vi "Auto Drive v2.vi"(9 "Orientation Angle":dbl, 10 "Move Distance":dbl, 11 "Movement Angle":dbl) -> (0 "Done Moving":bool)   [LabVIEW 2017]
uses:
  Robot Global Data.vi
  <vilib>/addons/control/pid/pid.llb/PID (DBL).vi
  <vilib>/addons/control/pid/NI_PID_pid.lvlib
panel:
  out "Last 25 Compare Values":bool[](array[boolean])
  out "Drive Speed":enum16{"Fast", "Slow", "Approach", "Stopping"}(ring)
  in  "Stopping Setpoint":dbl=0.1
  in  "Approach Setpoint":dbl=0.3
  in  "Slow Setpoint":dbl=0.5
  in  "Allowable Encoder Error":dbl=425.0
  out "Encoder Out":dbl
  in  "Encoder":dbl
  out "Drive Encoder Value":dbl(graph)
  out "output - Angle":dbl(graph)
  in  "PID gains - Angle":T1={"proportional gain (Kc)"=0.0012, "integral time (Ti, min)"=0.0, "derivative time (Td, min)"=0.0002} {"derivative time (Td, min)" step=0.001 format="%.5f"; "integral time (Ti, min)" step=0.001 format="%.5f"; "proportional gain (Kc)" step=0.001 format="%.5f"}
  # "Note: Setpoint Values\nare based on decimal\nprecentages. Ex. 80%\nwill be entered 0.8"
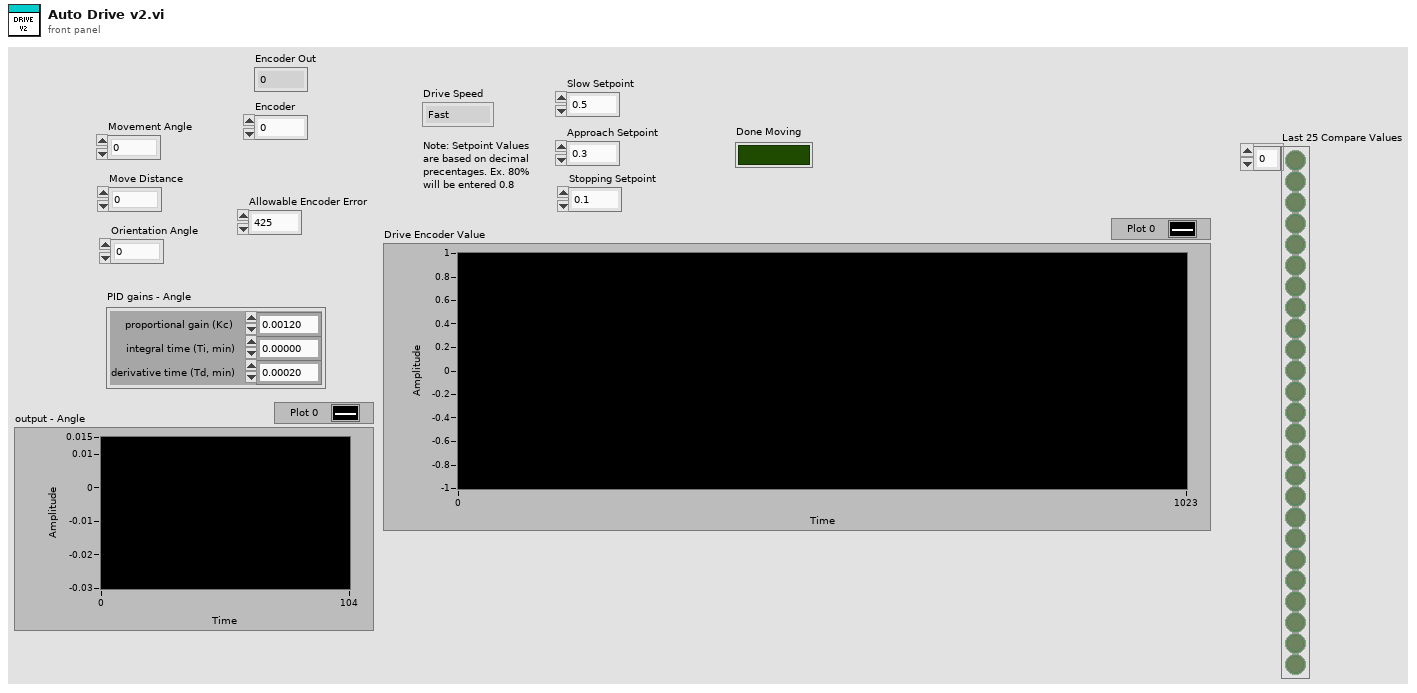
[diagram p1: front panel]
types:
  T1 = cluster{"proportional gain (Kc)":dbl, "integral time (Ti, min)":dbl, "derivative time (Td, min)":dbl}
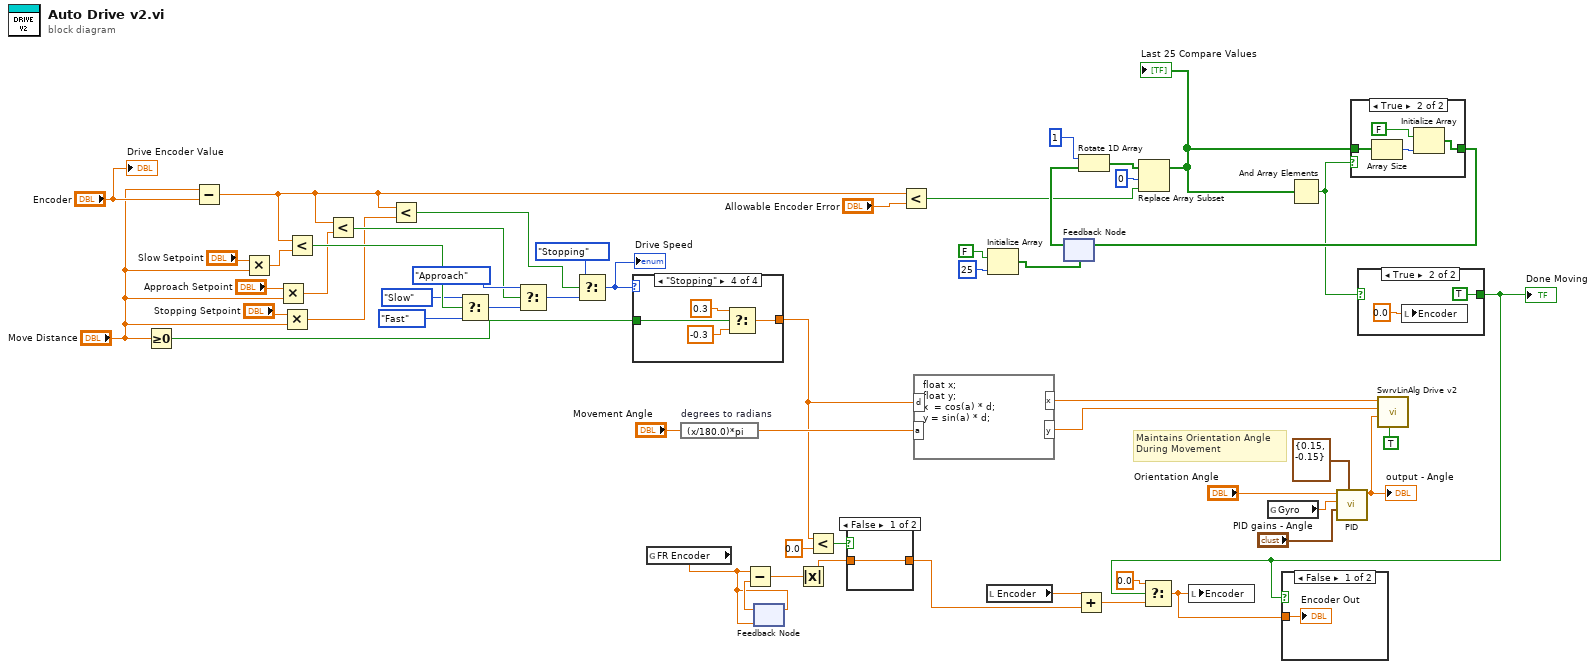
[diagram p0: block diagram]
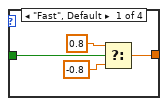
[diagram p2: hidden frame]
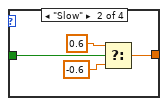
[diagram p3: hidden frame]
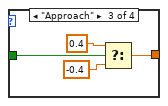
[diagram p4: hidden frame]
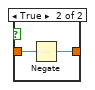
[diagram p7: hidden frame]
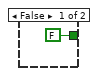
[diagram p8: hidden frame]
diagram:
  # "Maintains Orientation Angle\nDuring Movement"
  n1 = Greater Or Equal To 0?(x="Move Distance") -> (x >= 0?=w24:bool)
  n2 = Subtract(x="Move Distance", y="Encoder") -> (x-y=w1:dbl)
  n3 = Multiply(x="Slow Setpoint", y="Move Distance") -> (x*y=w14:dbl)
  n4 = Multiply(x="Approach Setpoint", y="Move Distance") -> (x*y=w10:dbl)
  n5 = Multiply(x="Stopping Setpoint", y="Move Distance") -> (x*y=w8:dbl)
  n6 = Less?(x=w1, y=w14) -> (x < y?=w21:bool)
  n7 = Less?(x=w1, y=w10) -> (x < y?=w12:bool)
  n8 = Less?(x=w1, y=w8) -> (x < y?=w13:bool)
  n9 = Select(t=enum16{"Fast", "Slow", "Approach", "Stopping"}."Slow", s=w21, f=enum16{"Fast", "Slow", "Approach", "Stopping"}."Fast" ("Drive Speed")) -> (s? t:f=w22:enum16{"Fast", "Slow", "Approach", "Stopping"})
  n10 = Select(t=enum16{"Fast", "Slow", "Approach", "Stopping"}."Approach", s=w12, f=w22) -> (s? t:f=w20:enum16{"Fast", "Slow", "Approach", "Stopping"})
  n11 = Select(t=enum16{"Fast", "Slow", "Approach", "Stopping"}."Stopping", s=w13, f=w20) -> (s? t:f=w16:enum16{"Fast", "Slow", "Approach", "Stopping"})
  "Drive Speed" <- w16
  n12 = case shown="\"Stopping\"" w16 {
    tunnel: w24 -> [w59 w63 w67 w71]
    tunnel: [w56 w60 w64 w68] -> w6
    frame "Fast", Default {
      n13 = Select(t=0.8, s=w59, f=-0.8) -> (s? t:f=w56:dbl)
    }
    frame "Slow" {
      n14 = Select(t=0.6, s=w63, f=-0.6) -> (s? t:f=w60:dbl)
    }
    frame "Approach" {
      n15 = Select(t=0.4, s=w67, f=-0.4) -> (s? t:f=w64:dbl)
    }
    frame "Stopping" {
      n16 = Select(t=0.3, s=w71, f=-0.3) -> (s? t:f=w68:dbl)
    }
  }
  n17 = global read "Robot Global Data.vi" "FR Encoder"() -> (w45:dbl)
  n18 = expression code="(x/180.0)*pi" "degrees to radians"("Movement Angle") -> (w32:dbl)
  n19 = feedback #1(w45) -> (w50:dbl)
  n20 = Subtract(x=w45, y=w50) -> (x-y=w49:dbl)
  n21 = feedback-in #1(w45) -> ()
  n22 = Absolute Value(x=w49) -> (abs(x)=w46:dbl)
  n23 = Less?(x=w6, y=0.0) -> (x < y?=w47:bool)
  n24 = case shown="False" w47 {
    tunnel: w46 -> [w72 w74]
    tunnel: [w72 w73] -> w29
    frame False {
    }
    frame True {
      n25 = Negate(x=w74) -> (-x=w73:dbl)
    }
  }
  n26 = Less?(x=w1, y="Allowable Encoder Error") -> (x < y?=w3:bool)
  n27 = formula code="float x;\nfloat y;\nx  = cos(a) * d;\ny = sin(a) * d;"("d"=w6, "a"=w32) -> ("x"=w30:dbl, "y"=w31:dbl)
  n28 = local read "Encoder"() -> (w43:dbl)
  n29 = Initialize Array(FALSE, 25 ("dimension size")) -> (w36:bool[])
  n30 = feedback #2(w36) -> (w38:bool[])
  n31 = Add(x=w43, y=w29) -> (x+y=w44:dbl)
  n32 = Rotate 1D Array(1:w38, 2:1 ("n")) -> (0:w40:bool[])
  n33 = Replace Array Subset(array=w40, new element=w3, index=0) -> (w5:bool[])
  "Last 25 Compare Values" <- w5
  n34 = global read "Robot Global Data.vi" "Gyro"() -> (w51:dbl)
  n35 = And Array Elements(Boolean array=w5) -> (logical AND=w33:bool)
  n36 = call-poly <vilib>:"PID.vi"("output range"=cluster{"output high":dbl, "output low":dbl} {"output high"=0.15, "output low"=-0.15}, "PID gains"="PID gains - Angle", "process variable"=w51, "setpoint"="Orientation Angle") -> ("output"=w26:dbl)  [unwired: 6 in, 1 out]
  "output - Angle" <- w26
  n37 = case shown="True" w33 {
    tunnel: w5 -> [w75 w77]
    tunnel: [w75 w76] -> w37
    frame False {
    }
    frame True {
      n38 = Array Size(array=w77) -> (size(s)=w78:i32)
      n39 = Initialize Array(FALSE, w78) -> (w76:bool[])
    }
  }
  n40 = feedback-in #2(w37) -> ()
  n41 = case shown="True" w33 {
    tunnel: [FALSE TRUE] -> w25
    frame False {
    }
    frame True {
      n42 = local write "Encoder"(0.0 ("Encoder")) -> ()
    }
  }
  "Done Moving" <- w25
  n43 = Select(t=0.0, s=w25, f=w44) -> (s? t:f=w27:dbl)
  n44 = local write "Encoder"(w27) -> ()
  n45 = case shown="False" w25 {
    tunnel: w27 -> [w83 _]
    frame False {
      "Encoder Out" <- w83
    }
    frame True {
    }
  }
  n46 = call "SwrvLinAlg Drive v2.vi"("Auto Controls"=TRUE, "Z"=w26, "Y"=w31, "X"=w30) -> ()  [unwired: 8 in]
  "Drive Encoder Value" <- "Encoder"
